vi "Fix Path.vi"(8 "error in (no error)":errorcluster, 10 "Request Path":string) -> (0 "error out":errorcluster, 2 "Fixed":string)   [LabVIEW 2023, in "Server.lvclass"]
uses:
  Server.lvclass
  Server.lvclass/Server.ctl
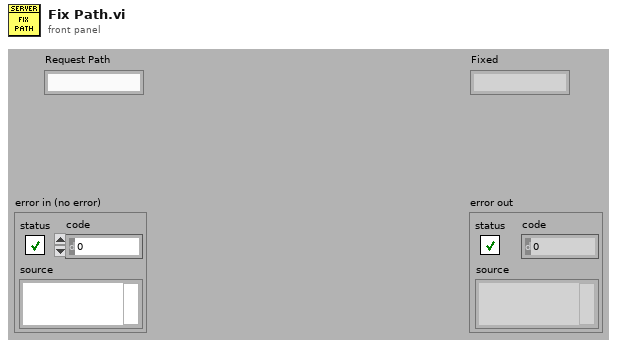
[diagram p1: front panel]
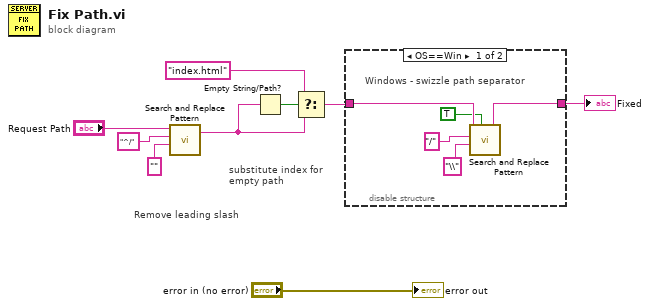
[diagram p0: block diagram]
diagram:
  # "substitute index for\nempty path"
  # "Remove leading slash"
  n1 = call <vilib>:"Search and Replace Pattern.vi"("string"="Request Path", "regular expression (\"\")"="^/" ("regular expression (\"\")"), "replace string (\"\")"="" ("regular expression (\"\")")) -> ("result string"=w3:string)  [unwired: 2 in, 1 out]
  n2 = Empty String/Path?(string/path=w3) -> (empty?=w5:bool)
  n3 = Select(t="index.html" ("regular expression (\"\")"), s=w5, f=w3) -> (s? t:f=w2:string)
  n4 = disable-structure shown="OS==Win" {
    disable-tunnel: w2 -> [w12 w15]
    disable-tunnel: [w11 w15] -> w1
    frame condition #0 (active) {
      # "Windows - swizzle path separator"
      n5 = call <vilib>:"Search and Replace Pattern.vi"("string"=w12, "regular expression (\"\")"="/" ("regular expression (\"\")"), "replace string (\"\")"="\\" ("regular expression (\"\")"), "replace all? (F)"=TRUE) -> ("result string"=w11:string)  [unwired: 1 in, 1 out]
    }
    frame condition #1 {
      # "Not Windows - path separator is fine"
    }
  }
  "Fixed" <- w1
  "error out" <- "error in (no error)"
